vi "Limits.vi"() -> ()   [LabVIEW 2015]
panel:
  out "output variable":dbl
  in  "input variable":dbl
  in  "low limit":dbl
  in  "high limit":dbl
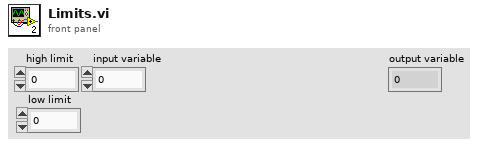
[diagram p1: front panel]
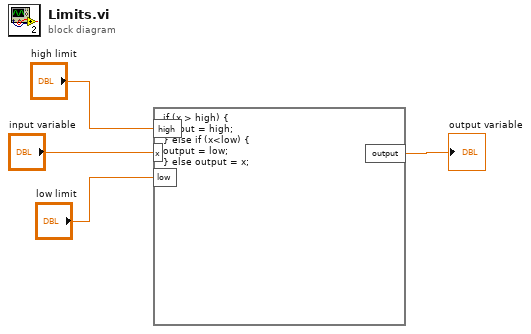
[diagram p0: block diagram]
diagram:
  n1 = formula code="if (x > high) {\noutput = high;\n} else if (x<low) {\noutput = low;\n} else output = x;"("high"="high limit", "low"="low limit", "x"="input variable") -> ("output"=→"output variable":dbl)
